vi "Begin.vi"(8 "error in":errorcluster) -> (0 "error out":errorcluster)   [LabVIEW 2020]
doc: "Called before other user functions, this VI is expected to open initial I/O refnums, load in file data, and do all program initialization. Notice that the <B>error out</B> terminal is simply used for data flow. Wiring it to other structures or subVIs ensures that this VI runs first."
uses:
  <vilib>/Rock Robotics/WPI/DriverStation/WPI_DriverStationRobotMode2.ctl
  <vilib>/Rock Robotics/WPI/Joystick/WPI_JoystickDeviceEnum.ctl
  <vilib>/Rock Robotics/WPI/SafetyOutput/WPI_SafetyOutputConfigMenu.ctl
  Robot Global Data.vi
  <vilib>/Rock Robotics/Network Tables/NT Write String Array.vi
  <vilib>/Rock Robotics/SystemInterfaces/DIO/FPGA_DIOPWMChannel.ctl
  <vilib>/Rock Robotics/WPI/RobotDrive/WPI_RobotDriveOpen2MotorWithVictorSPX.vi
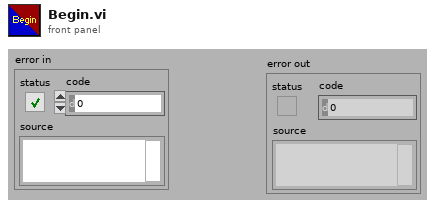
[diagram p1: front panel]
types:
  T1 = typedef "WPI_SafetyOutputConfigMenu.ctl" = enum16{"Enable", "Disable"}
  T2 = typedef "WPI_JoystickDeviceEnum.ctl" = enum16{"USB 0", "USB 1", "USB 2", "USB 3", "USB 4", "USB 5"}
  T3 = typedef "WPI_DriverStationRobotMode2.ctl" = enum16{"Autonomous Disabled", "Autonomous Enabled", "Teleop Disabled", "Teleop Enabled", "Disconnected", "Finish", "Test Disabled", "Test Enabled", "Emergency Stopped"}
  T4 = typedef "WPI_MotorControlDeviceRef.ctl" = cluster{"DeviceStatus":errorcluster, "Type":T5, "PWM":cluster{"PWM Channel":T6, "DeadBand":T7}, "CAN":cluster{"Device Number":u8, "SetOutput VI Ref":variant, "GetOutput VI Ref":variant, "Enable VI Ref":variant, "Disable VI Ref":variant, "Data":variant}, "Invert":bool, "DIO PWM":cluster{"PWM \"Enable\" Channel":T6, "DIOChannel":T8, "PWM Rate":dbl}}
  T5 = typedef "WPI_MotorControlType.ctl" = enum16{"PWM", "CAN", "DIO PWM"}
  T6 = typedef "FPGA_DIOPWMChannel.ctl" = enum8{"PWM 0", "PWM 1", "PWM 2", "PWM 3", "PWM 4", "PWM 5", "PWM 6", "PWM 7", "PWM 8", "PWM 9", "PWM MXP 0", "PWM MXP 1", "PWM MXP 2", "PWM MXP 3", "PWM MXP 4", "PWM MXP 5", "PWM MXP 6", "PWM MXP 7", "PWM MXP 8", "PWM MXP 9", "Invalid"}
  T7 = typedef "WPI_PWMDeadband.ctl" = cluster{"Name":string, "maxPositivePwm":i32, "minPositivePwm":i32, "centerPwm":i32, "maxNegativePwm":i32, "minNegativePwm":i32, "angularRange":u16}
  T8 = typedef "FPGA_DIOChannel.ctl" = enum8{"DIO 0", "DIO 1", "DIO 2", "DIO 3", "DIO 4", "DIO 5", "DIO 6", "DIO 7", "DIO 8", "DIO 9", "DIO MXP 0", "DIO MXP 1", "DIO MXP 2", "DIO MXP 3", "DIO MXP 4", "DIO MXP 5", "DIO MXP 6", "DIO MXP 7", "DIO MXP 8", "DIO MXP 9", "DIO MXP 10", "DIO MXP 11", "DIO MXP 12", "DIO MXP 13", "DIO MXP 14", "DIO MXP 15", "SPI Port CS1", "SPI Port CS2", "SPI Port CS3", "SPI Port MISO", "SPI Port MOSI", "Invalid"}
  T9 = typedef "WPI_RobotDriveDevRef.ctl" = cluster{"DevStatus":errorcluster, "Motors[]":T4[], "Square Inputs":bool, "Max Output":dbl}
  T10 = typedef "ADIS16470 Device Reference.ctl" = cluster{"DevStatus":errorcluster, "Hardware Config":T11, "Calibration Complete":refnum<notifier>, "Status Reference":refnum<data-value>, "Data Reference":refnum<data-value>, "Sychronous Process VI":T14, "Cmd FIFO":refnum<k33>, "Source":T15, "Data FIFO":refnum<k33>, "Calibration Time (ms)":u32, "Data Reference":refnum<data-value>}
  T11 = typedef "ADIS16470 Hardware Configuration.ctl" = cluster{"SPI Clock Rate (Hz)":dbl, "IMU SPI Mode (3)":T12, "IMU Reset Pin":T8, "IMU SPI Bus":T13, "IMU Data Ready Pin":T8, "Stall Config":cluster{"Pow2BytesPerRead":u8, "StallTicks":u16, "CsToSclkTicks":u8}}
  T12 = typedef "WPI_SPIMode.ctl" = enum16{"Mode 0 (Clk Idle Low,Sample on Leading)", "Mode 1 (Clk Idle Low,Sample on Trailing)", "Mode 2 (Clk Idle High,Sample on Leading)", "Mode 3 (Clk Idle High,Sample on Trailing)"}
  T13 = typedef "spi_bus.ctl" = enum16{"SPI On-Board, CS0", "SPI On-Board, CS1", "SPI On-Board, CS2", "SPI On-Board, CS3", "SPI MXP", "Invalid"}
  T14 = typedef "ADIS16470 Process.ctl" = refnum<vi>
  T15 = typedef "FPGA_CounterEncoderSourceConvertionLVSourceType.ctl" = cluster{"DevStatus":errorcluster, "AnalogTriggerMode?":bool, "DigitalMode":cluster{"DIO Channel":T16}, "AnalogTriggerMode":cluster{"AnalogTriggerIndex":T17, "OutputType":T18}}
  T16 = typedef "FPGA_DIODigitalSourceChannel.ctl" = enum8{"DIO 0", "DIO 1", "DIO 2", "DIO 3", "DIO 4", "DIO 5", "DIO 6", "DIO 7", "DIO 8", "DIO 9", "DIO MXP 0", "DIO MXP 1", "DIO MXP 2", "DIO MXP 3", "DIO MXP 4", "DIO MXP 5", "DIO MXP 6", "DIO MXP 7", "DIO MXP 8", "DIO MXP 9", "DIO MXP 10", "DIO MXP 11", "DIO MXP 12", "DIO MXP 13", "DIO MXP 14", "DIO MXP 15", "SPI Port CS1", "SPI Port CS2", "SPI Port CS3", "SPI Port MISO", "SPI Port MOSI", "Disabled"}
  T17 = typedef "FPGA_AnalogTriggerIndex.ctl" = enum8{"Trig 0", "Trig 1", "Trig 2", "Trig 3", "Trig 4", "Trig 5", "Trig 6", "Trig 7", "Invalid"}
  T18 = typedef "FPGA_AnalogTriggerOutType.ctl" = enum16{"InWindow", "TriggerState", "Rising", "Falling"}
  T19 = typedef "WPI_JoystickDevRef.ctl" = cluster{"Device":T2}
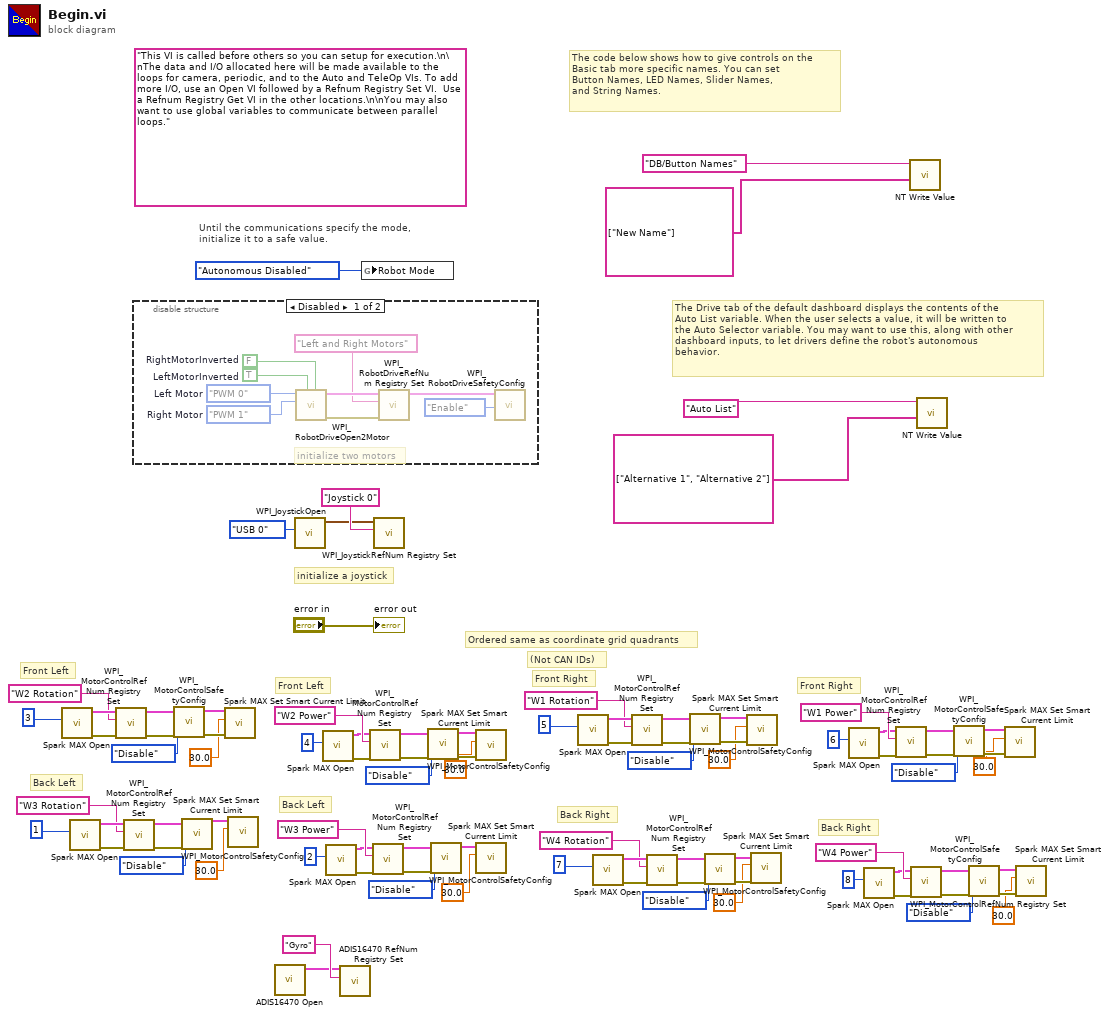
[diagram p0: block diagram]
diagram:
  (unwired) "This VI is called before others so you can setup for execution.\n\nThe data and I/O allocated here will be made available to the loops for camera, periodic, and to the Auto and TeleOp VIs. To add more I/O, use an Open VI followed by a Refnum Registry Set VI.  Use a Refnum Registry Get VI in the other locations.\n\nYou may also want to use global variables to communicate between parallel loops."
  # "(Not CAN IDs)"
  # "Ordered same as coordinate grid quadrants"
  # "Back Right"
  # "Back Right"
  # "Back Left"
  # "Back Left"
  # "Front Left"
  # "Front Left"
  # "Front Right"
  # "Front Right"
  # "The Drive tab of the default dashboard displays the contents of the\nAuto List variable. When the user selects a value, it will be written to\nthe Auto Selector variable. You may want to use this, along with other\ndashboard inputs, to let drivers define the robot's autonomous\nbehavior."
  # "The code below shows how to give controls on the\nBasic tab more specific names. You can set\nButton Names, LED Names, Slider Names,\nand String Names."
  # "initialize a joystick"
  # "Until the communications specify the mode,\ninitialize it to a safe value."
  n1 = call <vilib>:"Spark MAX Open.vi"("Device Number"=u8 3) -> ("error out"=w67:errorcluster, "MotorControlDeviceRef"=w66:T4)  [unwired: 9 in]
  n2 = call <vilib>:"Spark MAX Open.vi"("Device Number"=u8 1) -> ("error out"=w54:errorcluster, "MotorControlDeviceRef"=w53:T4)  [unwired: 9 in]
  n3 = call <vilib>:"WPI_MotorControlRefNum Registry Set.vi"("error in (no error)"=w67, "refnum name"="W2 Rotation", "MotorControlDevRef"=w66) -> ("error out"=w65:errorcluster, "MotorControlDevRef"=w64:T4)  [unwired: 7 in]
  n4 = call <vilib>:"WPI_MotorControlRefNum Registry Set.vi"("error in (no error)"=w54, "refnum name"="W3 Rotation", "MotorControlDevRef"=w53) -> ("error out"=w52:errorcluster, "MotorControlDevRef"=w51:T4)  [unwired: 7 in]
  n5 = disable-structure shown="Disabled" {
    frame Disabled {
      w92 = FPGA_DIOPWMChannel."PWM 1"  # Right Motor
      w93 = FPGA_DIOPWMChannel."PWM 0"  # Left Motor
      w97 = TRUE  # LeftMotorInverted
      w98 = FALSE  # RightMotorInverted
      # "initialize two motors"
      n6 = call-poly <vilib>:"WPI_RobotDriveOpen2Motor.vi"("Right Motor Inverted"=w98, "Left Motor Inverted"=w97, "Right Motor"=w92, "Left Motor"=w93) -> ("error out"=w94:errorcluster, "RobotDriveDevRef"=w96:T9)  [unwired: 1 in, 5 out]
      n7 = call <vilib>:"WPI_RobotDriveRefNum Registry Set.vi"("error in (no error)"=w94, "refnum name"="Left and Right Motors", "RobotDriveDevRef"=w96) -> ("RobotDriveDevRef"=w91:T9)  [unwired: 1 in, 7 out]
      n8 = call <vilib>:"WPI_RobotDriveSafetyConfig.vi"("mode"=WPI_SafetyOutputConfigMenu."Enable", "RobotDriveDevRef"=w91) -> ()  [unwired: 8 in, 2 out]
    }
    frame Enabled {
    }
  }
  n9 = call <vilib>:"WPI_MotorControlSafetyConfig.vi"("error in (no error)"=w65, "mode"=WPI_SafetyOutputConfigMenu."Disable", "MotorControlDevRef"=w64) -> ("error out"=w3:errorcluster, "MotorControlDevRef"=w2:T4)  [unwired: 7 in]
  n10 = call <vilib>:"WPI_MotorControlSafetyConfig.vi"("error in (no error)"=w52, "mode"=WPI_SafetyOutputConfigMenu."Disable", "MotorControlDevRef"=w51) -> ("MotorControlDevRef"=w22:T4)  [unwired: 7 in, 1 out]
  n11 = call <vilib>:"Spark MAX Set Smart Current Limit.vi"("error in (no error)"=w3, "Primay Current Limit (80A)"=30.0, "MotorControlDeviceRef in"=w2) -> ()  [unwired: 7 in, 2 out]
  n12 = call <vilib>:"Spark MAX Set Smart Current Limit.vi"("Primay Current Limit (80A)"=30.0, "MotorControlDeviceRef in"=w22) -> ()  [unwired: 8 in, 2 out]
  n13 = call <vilib>:"ADIS16470 Open.vi"() -> ("ADIS16470DevRef"=w23:T10)  [unwired: 10 in, 1 out]
  n14 = call <vilib>:"WPI_JoystickOpen.vi"("JoystickDevice"=WPI_JoystickDeviceEnum."USB 0") -> ("JoystickDevRef"=w87:T19)  [unwired: 10 in]
  n15 = call <vilib>:"Spark MAX Open.vi"("Device Number"=u8 4) -> ("error out"=w56:errorcluster, "MotorControlDeviceRef"=w57:T4)  [unwired: 9 in]
  n16 = call <vilib>:"Spark MAX Open.vi"("Device Number"=u8 2) -> ("error out"=w43:errorcluster, "MotorControlDeviceRef"=w44:T4)  [unwired: 9 in]
  n17 = call <vilib>:"ADIS16470 RefNum Registry Set.vi"("refnum name"="Gyro", "ADIS16470DevRef in"=w23) -> ()  [unwired: 8 in, 2 out]
  n18 = global write "Robot Global Data.vi" "Robot Mode"(WPI_DriverStationRobotMode2."Autonomous Disabled" ("Robot Mode")) -> ()
  n19 = call <vilib>:"WPI_MotorControlRefNum Registry Set.vi"("error in (no error)"=w56, "refnum name"="W2 Power", "MotorControlDevRef"=w57) -> ("error out"=w61:errorcluster, "MotorControlDevRef"=w60:T4)  [unwired: 7 in]
  n20 = call <vilib>:"WPI_MotorControlRefNum Registry Set.vi"("error in (no error)"=w43, "refnum name"="W3 Power", "MotorControlDevRef"=w44) -> ("error out"=w48:errorcluster, "MotorControlDevRef"=w47:T4)  [unwired: 7 in]
  n21 = call <vilib>:"WPI_JoystickRefNum Registry Set.vi"("refnum name"="Joystick 0", "JoystickDevRef"=w87) -> ()  [unwired: 8 in, 2 out]
  n22 = call <vilib>:"WPI_MotorControlSafetyConfig.vi"("error in (no error)"=w61, "mode"=WPI_SafetyOutputConfigMenu."Disable", "MotorControlDevRef"=w60) -> ("error out"=w6:errorcluster, "MotorControlDevRef"=w5:T4)  [unwired: 7 in]
  n23 = call <vilib>:"WPI_MotorControlSafetyConfig.vi"("error in (no error)"=w48, "mode"=WPI_SafetyOutputConfigMenu."Disable", "MotorControlDevRef"=w47) -> ("MotorControlDevRef"=w20:T4)  [unwired: 7 in, 1 out]
  n24 = call <vilib>:"Spark MAX Set Smart Current Limit.vi"("error in (no error)"=w6, "Primay Current Limit (80A)"=30.0, "MotorControlDeviceRef in"=w5) -> ()  [unwired: 7 in, 2 out]
  n25 = call <vilib>:"Spark MAX Set Smart Current Limit.vi"("Primay Current Limit (80A)"=30.0, "MotorControlDeviceRef in"=w20) -> ()  [unwired: 8 in, 2 out]
  n26 = call <vilib>:"Spark MAX Open.vi"("Device Number"=u8 5) -> ("error out"=w80:errorcluster, "MotorControlDeviceRef"=w79:T4)  [unwired: 9 in]
  n27 = call <vilib>:"Spark MAX Open.vi"("Device Number"=u8 7) -> ("error out"=w41:errorcluster, "MotorControlDeviceRef"=w40:T4)  [unwired: 9 in]
  n28 = call <vilib>:"WPI_MotorControlRefNum Registry Set.vi"("error in (no error)"=w80, "refnum name"="W1 Rotation", "MotorControlDevRef"=w79) -> ("error out"=w78:errorcluster, "MotorControlDevRef"=w77:T4)  [unwired: 7 in]
  n29 = call <vilib>:"WPI_MotorControlRefNum Registry Set.vi"("error in (no error)"=w41, "refnum name"="W4 Rotation", "MotorControlDevRef"=w40) -> ("error out"=w39:errorcluster, "MotorControlDevRef"=w38:T4)  [unwired: 7 in]
  n30 = call <vilib>:"WPI_MotorControlSafetyConfig.vi"("error in (no error)"=w78, "mode"=WPI_SafetyOutputConfigMenu."Disable", "MotorControlDevRef"=w77) -> ("error out"=w9:errorcluster, "MotorControlDevRef"=w8:T4)  [unwired: 7 in]
  n31 = call <vilib>:"WPI_MotorControlSafetyConfig.vi"("error in (no error)"=w39, "mode"=WPI_SafetyOutputConfigMenu."Disable", "MotorControlDevRef"=w38) -> ("error out"=w18:errorcluster, "MotorControlDevRef"=w17:T4)  [unwired: 7 in]
  n32 = call <vilib>:"Spark MAX Set Smart Current Limit.vi"("error in (no error)"=w9, "Primay Current Limit (80A)"=30.0, "MotorControlDeviceRef in"=w8) -> ()  [unwired: 7 in, 2 out]
  n33 = call <vilib>:"Spark MAX Set Smart Current Limit.vi"("error in (no error)"=w18, "Primay Current Limit (80A)"=30.0, "MotorControlDeviceRef in"=w17) -> ()  [unwired: 7 in, 2 out]
  n34 = call <vilib>:"Spark MAX Open.vi"("Device Number"=u8 6) -> ("error out"=w69:errorcluster, "MotorControlDeviceRef"=w70:T4)  [unwired: 9 in]
  n35 = call <vilib>:"Spark MAX Open.vi"("Device Number"=u8 8) -> ("error out"=w30:errorcluster, "MotorControlDeviceRef"=w31:T4)  [unwired: 9 in]
  n36 = call <vilib>:"WPI_MotorControlRefNum Registry Set.vi"("error in (no error)"=w69, "refnum name"="W1 Power", "MotorControlDevRef"=w70) -> ("error out"=w74:errorcluster, "MotorControlDevRef"=w73:T4)  [unwired: 7 in]
  n37 = call-poly <vilib>:"NT Write Value.vi"("String Array"=string[] ["New Name"], "Name"="DB/Button Names") -> ()  [unwired: 9 in, 1 out]
  n38 = call <vilib>:"WPI_MotorControlRefNum Registry Set.vi"("error in (no error)"=w30, "refnum name"="W4 Power", "MotorControlDevRef"=w31) -> ("error out"=w35:errorcluster, "MotorControlDevRef"=w34:T4)  [unwired: 7 in]
  n39 = call-poly <vilib>:"NT Write Value.vi"("String Array"=string[] ["Alternative 1", "Alternative 2"], "Name"="Auto List") -> ()  [unwired: 9 in, 1 out]
  n40 = call <vilib>:"WPI_MotorControlSafetyConfig.vi"("error in (no error)"=w74, "mode"=WPI_SafetyOutputConfigMenu."Disable", "MotorControlDevRef"=w73) -> ("error out"=w12:errorcluster, "MotorControlDevRef"=w11:T4)  [unwired: 7 in]
  n41 = call <vilib>:"WPI_MotorControlSafetyConfig.vi"("error in (no error)"=w35, "mode"=WPI_SafetyOutputConfigMenu."Disable", "MotorControlDevRef"=w34) -> ("error out"=w15:errorcluster, "MotorControlDevRef"=w14:T4)  [unwired: 7 in]
  n42 = call <vilib>:"Spark MAX Set Smart Current Limit.vi"("error in (no error)"=w12, "Primay Current Limit (80A)"=30.0, "MotorControlDeviceRef in"=w11) -> ()  [unwired: 7 in, 2 out]
  n43 = call <vilib>:"Spark MAX Set Smart Current Limit.vi"("error in (no error)"=w15, "Primay Current Limit (80A)"=30.0, "MotorControlDeviceRef in"=w14) -> ()  [unwired: 7 in, 2 out]
  "error out" <- "error in"
